vi "DAC Run.vi"(8 "error in":errorcluster, 11 "DAC Shunt dU in":refnum<class "DAC Heater dU.lvclass">) -> (0 "error out":errorcluster, 3 "DAC Heater dU out":refnum<class "DAC Heater dU.lvclass">)   [LabVIEW 2019, in "DAC.lvlib" / "DAC Heater dU.lvclass"]
uses:
  DAC Heater dU.lvclass
  C:/Users/wg/Documents/LV_Projects/TestStand/App/DAC/DAC.lvclass
  DAC.lvclass/DAC.ctl
  Results/LNG Boiling Results/LNG Boiling Results.lvclass
  Results/Results Method.ctl
  DAC Heater dU.lvclass/DAC Heater dU.ctl
  Results/LNG Boiling Results/LNG Boiling Results.lvclass/LNG Boiling Results.ctl
  <vilib>/DAQmx/read.llb/DAQmx Read (Analog DBL 1Chan 1Samp).vi
  <vilib>/DAQmx/miscellaneous.llb/DAQmx Fill In Error Info.vi
  DAC.lvclass
  Results/Results.lvlib
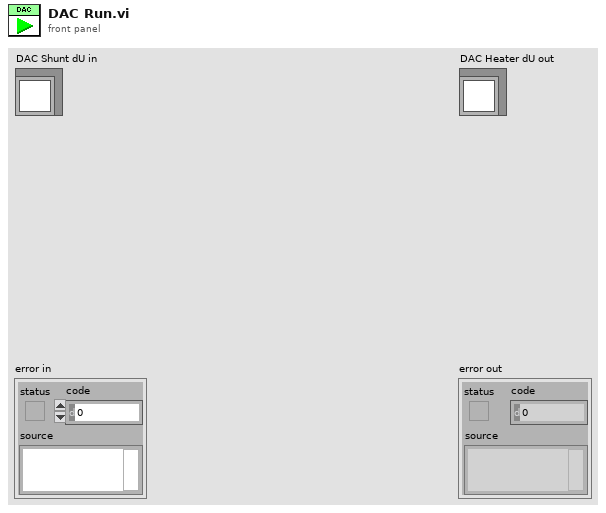
[diagram p1: front panel]
types:
  T1 = typedef "Results.lvlib/Results Method.ctl" = enum16{"Get", "Set"}
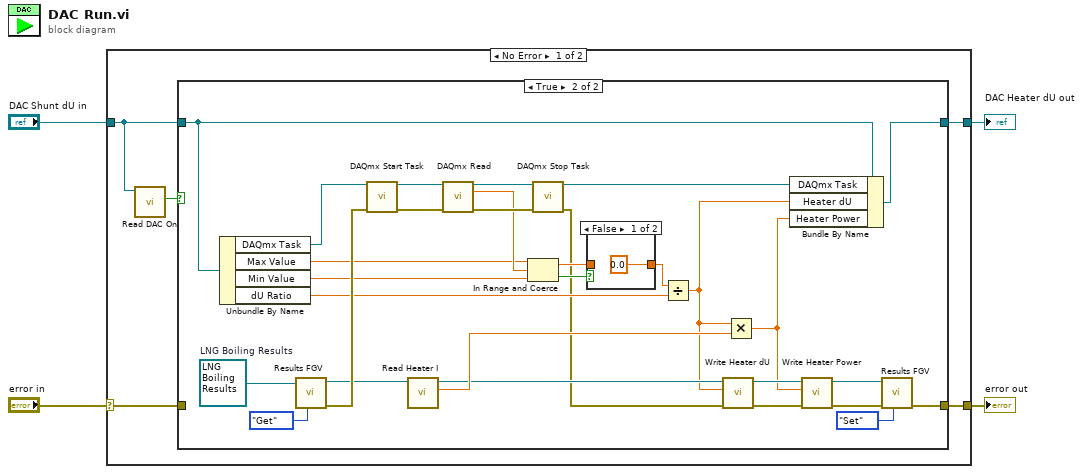
[diagram p0: block diagram]
diagram:
  n1 = case shown="No Error" "error in" {
    selector: "error in" -> [w7 w45]
    tunnel: [w6 w45] -> w2
    tunnel: [w8 w44] -> w1
    tunnel: "DAC Shunt dU in" -> [w5 w44]
    frame No Error {
      n2 = call "Read DAC On.vi"("DAC in"=w5) -> ("DAC On"=w9:bool)  [unwired: 8 in, 2 out]
      n3 = case shown="True" w9 {
        tunnel: w5 -> [w11 w37]
        tunnel: [w11 w30] -> w8
        tunnel: w7 -> [w10 _]
        tunnel: [w10 w29] -> w6
        frame False {
        }
        frame True {
          w36 = refnum<class "LNG Boiling Results.lvclass"> refnum  # LNG Boiling Results
          n4 = Unbundle By Name(w37) -> ("DAQmx Task"=w41:refnum<k21>, "Max Value"=w23:dbl, "Min Value"=w24:dbl, "dU Ratio"=w26:dbl)
          n5 = call-dynamic "Results FGV.vi"("Method"=Results_Method."Get", "LNG Boiling Results in"=w36) -> ("error out"=w33:errorcluster, "LNG Boiling Results out"=w28:refnum<class "LNG Boiling Results.lvclass">)  [unwired: 8 in]
          n6 = call <vilib>:"DAQmx Start Task.vi"("task/channels in"=w41, "error in"=w33) -> ("task out"=w40:refnum<k21>, "error out"=w39:errorcluster)  [unwired: 12 in]
          n7 = call "Read Heater I.vi"("LNG Boiling Results in"=w28) -> ("Heater I"=w27:dbl, "LNG Boiling Results out"=w20:refnum<class "LNG Boiling Results.lvclass">)  [unwired: 8 in, 1 out]
          n8 = call-poly <vilib>:"DAQmx Read.vi"("task/channels in"=w40, "error in"=w39) -> ("task out"=w31:refnum<k21>, "data"=w25:dbl, "error out"=w38:errorcluster)  [unwired: 11 in]
          n9 = In Range and Coerce(upper limit=w23, x=w25, lower limit=w24) -> (coerced(x)=w21:dbl, In Range?=w22:bool)
          n10 = call <vilib>:"DAQmx Stop Task.vi"("task/channels in"=w31, "error in"=w38) -> ("task out"=w32:refnum<k21>, "error out"=w17:errorcluster)  [unwired: 12 in]
          n11 = case shown="False" w22 {
            tunnel: w21 -> [_ w43]
            tunnel: [0.0 ("Max Value") w43] -> w16
            frame False {
            }
            frame True {
            }
          }
          n12 = Divide(x=w16, y=w26) -> (x/y=w15:dbl)
          n13 = call "Write Heater dU.vi"("error in (no error)"=w17, "Heater dU"=w15, "LNG Boiling Results in"=w20) -> ("error out"=w13:errorcluster, "LNG Boiling Results out"=w19:refnum<class "LNG Boiling Results.lvclass">)  [unwired: 7 in]
          n14 = Multiply(x=w15, y=w27) -> (x*y=w14:dbl)
          n15 = Bundle By Name(cluster=w37, "DAQmx Task"=w32, "Heater dU"=w15, "Heater Power"=w14) -> (w30:refnum<class "DAC Heater dU.lvclass">)
          n16 = call "Write Heater Power.vi"("error in (no error)"=w13, "Heater Power"=w14, "LNG Boiling Results in"=w19) -> ("error out"=w12:errorcluster, "LNG Boiling Results out"=w18:refnum<class "LNG Boiling Results.lvclass">)  [unwired: 7 in]
          n17 = call-dynamic "Results FGV.vi"("Method"=Results_Method."Set", "error in"=w12, "LNG Boiling Results in"=w18) -> ("error out"=w29:errorcluster)  [unwired: 7 in, 1 out]
        }
      }
    }
    frame Error {
    }
  }
  "error out" <- w2
  "DAC Heater dU out" <- w1
